vi "cast.to.network.stream.vi"(11 "Test Case":T2={"data.valid"=FALSE, "data"={"enabled"=[FALSE, FALSE, FALSE, FALSE, FALSE, FALSE, FALSE, FALSE], "byte"=[0, 0, 0, 0, 0, 0, 0, 0]}, "buffer"=[0, 0, 0, 0, 0, 0, 0, 0, 0], "buffer.length"=0, "exp.buffer.value.1"=0, "index 1"=0, "exp.buffer.value.2"=0, "index 2"=0, "exp.buffer.length"=0} {"exp.buffer.value.2" format="%.0x"; "exp.buffer.value.1" format="%.0x"; "buffer" format="%.0x"; "data"."byte" format="%.0x"}) -> (3 "network Data Stream.ctl":cluster{"reset":bool, "Data Stream":T1})   [LabVIEW 2020]
uses:
  buffer.test.case.ctl
  data.ctl
  <instrlib>/_niInstr/Network/Ethernet/Utility/v1/FPGA/Network Data Stream.ctl
  <instrlib>/_niInstr/Network/Ethernet/Utility/v1/FPGA/niInstr Ethernet Utilities FPGA v1.lvlib
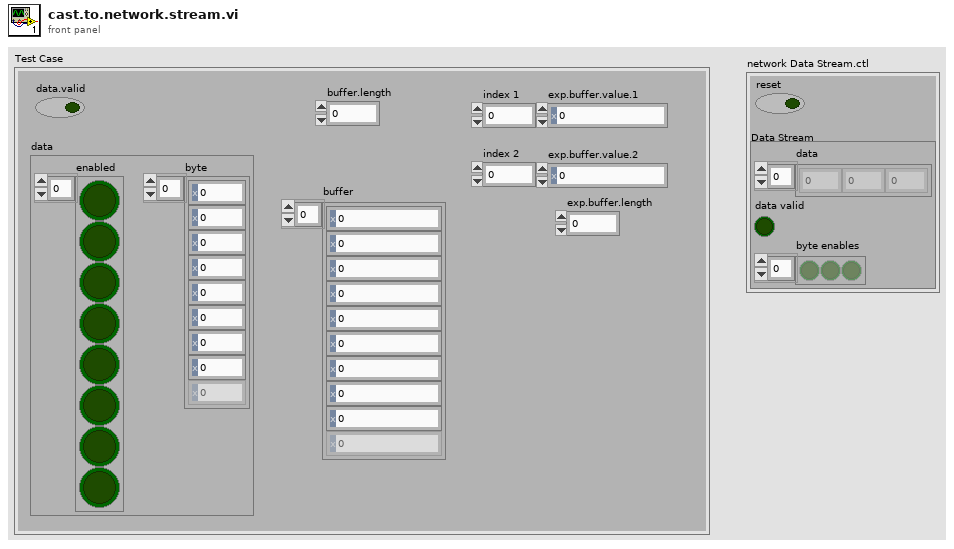
[diagram p1: front panel]
types:
  T1 = typedef "niInstr Ethernet Utilities FPGA v1.lvlib/Network Data Stream.ctl" = cluster{"data":u8[], "data valid":bool, "byte enables":bool[]}
  T2 = typedef "buffer.test.case.ctl" = cluster{"data.valid":bool, "data":T3, "buffer":u64[], "buffer.length":u8, "exp.buffer.value.1":u64, "index 1":i16, "exp.buffer.value.2":u64, "index 2":i16, "exp.buffer.length":u8}
  T3 = typedef "data.ctl" = cluster{"enabled":bool[], "byte":u8[]}
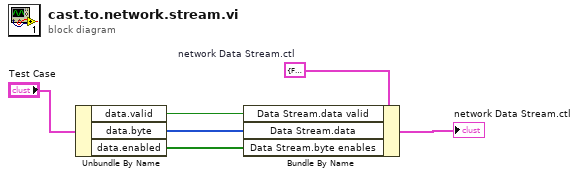
[diagram p0: block diagram]
diagram:
  w1 = cluster{"reset":bool, "Data Stream":T1} {"reset"=FALSE, "Data Stream"={"data"=[], "data valid"=FALSE, "byte enables"=[]}}  # network Data Stream.ctl
  n1 = Unbundle By Name("Test Case") -> ("data.valid"=w3:bool, "data.byte"=w4:u8[], "data.enabled"=w5:bool[])
  n2 = Bundle By Name(cluster=w1, "Data Stream.data valid"=w3, "Data Stream.data"=w4, "Data Stream.byte enables"=w5) -> (→"network Data Stream.ctl":cluster{"reset":bool, "Data Stream":T1})
